vi "Simulated tractor.vi"(2 "Angle":dbl(slide) scale=-180.0..180.0, 3 "Speed":dbl(slide) scale=-10.0..10.0) -> (0 "y out":dbl, 1 "x out":dbl)   [LabVIEW 2021]
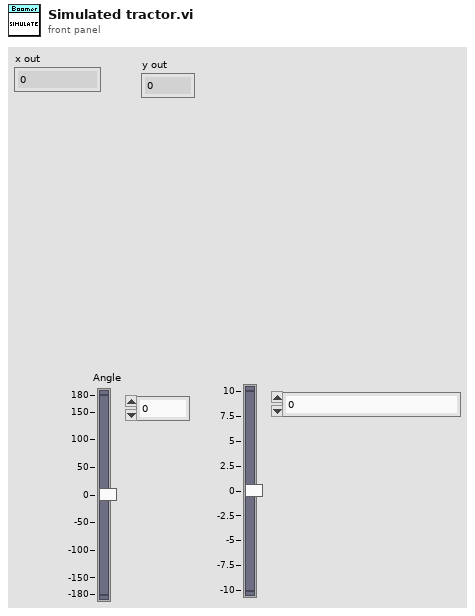
[diagram p1: front panel]
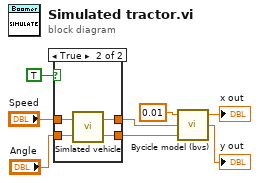
[diagram p0: block diagram]
diagram:
  n1 = case shown="True" TRUE {
    tunnel: "Speed" -> [w10 w14]
    tunnel: "Angle" -> [w9 w13]
    tunnel: [w10 w12] -> w5
    tunnel: [w9 w11] -> w1
    frame False {
    }
    frame True {
      n2 = call "Simlated vehicle.vi"("Steering angle"=w13, "Speed"=w14) -> ("Steering angle sensor"=w11:dbl, "Speed sensor"=w12:dbl)
    }
  }
  n3 = call "Bycicle model (bvs).vi"("Wheel angle (deg)"=w1, "Ground speed (km/h)"=w5, "dt (s)"=0.01 ("dt(s)")) -> ("New position Y"=→"y out":dbl, "New position X"=→"x out":dbl)  [unwired: 1 out]
